vi "ones.vi"   [LabVIEW 2017, in "NI_Gmath.lvlib"]
uses:
  <vilib>/gmath/NI_Gmath.lvlib
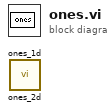
[diagram p0: block diagram]
diagram:
  n1 = call <vilib>:"ones_2d.vi"() -> ()  [unwired: 8 in, 1 out]
  n2 = call <vilib>:"ones_1d.vi"() -> ()  [unwired: 8 in, 1 out]
